vi "H5Lget_val (Soft).vi"(6 "lapl_id":T2, 8 "error in (no error)":errorcluster, 10 "Name":string=".", 11 "Location Ref":T2) -> (0 "error out":errorcluster, 1 "Object Path":string, 3 "Location Ref out":T2, 4 "type":T1 items=["H5L_TYPE_ERROR"=-1, "H5L_TYPE_HARD"=0, "H5L_TYPE_SOFT"=1, "H5L_TYPE_EXTERNAL"=64, "H5L_TYPE_MAX"=255])   [LabVIEW 2017]
doc: "Returns the value of a symbolic link."
uses:
  <vilib>/UPVI/lvhdf5/library.llb/HDF5 Ref.ctl
  <vilib>/UPVI/lvhdf5/link.llb/H5L_type_t.ctl
  <vilib>/UPVI/lvhdf5/error.llb/LVH5EMajorID.ctl
  <vilib>/UPVI/lvhdf5/error.llb/LVH5EMinorID.ctl
  <vilib>/UPVI/lvhdf5/error.llb/H5Epush_enum_enum.vi
panel:
  # "LVHDF5 Toolkit\nCopyright (c) 2005-2013 by Jason D. Sommerville\nCopyright (c) 2014-2015 by UPVI, LLC.\n\nThis use and distribution of this file is governed by the terms found in \nLICENSE.txt distributed with this toolkit and installed at\n <user.lib>\\_lvhdf5\\LICENSE.txt"
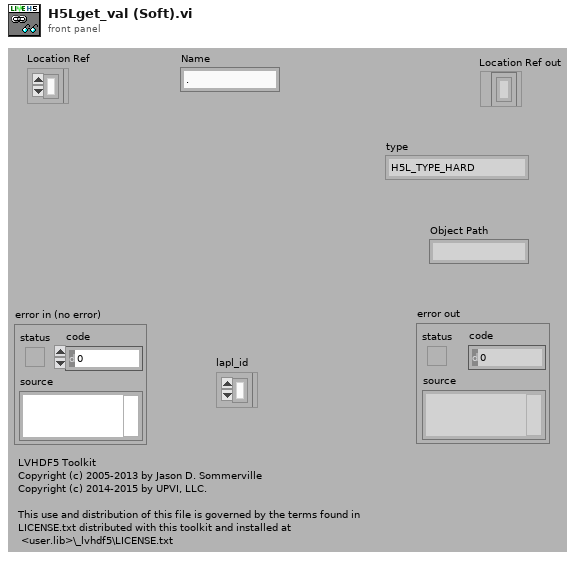
[diagram p1: front panel]
types:
  T1 = typedef "H5L_type_t.ctl" = i32
  T2 = typedef "HDF5 Ref.ctl" = refnum<k1>
  T3 = typedef "LVH5EMinorID.ctl" = string
  T4 = typedef "LVH5EMajorID.ctl" = string
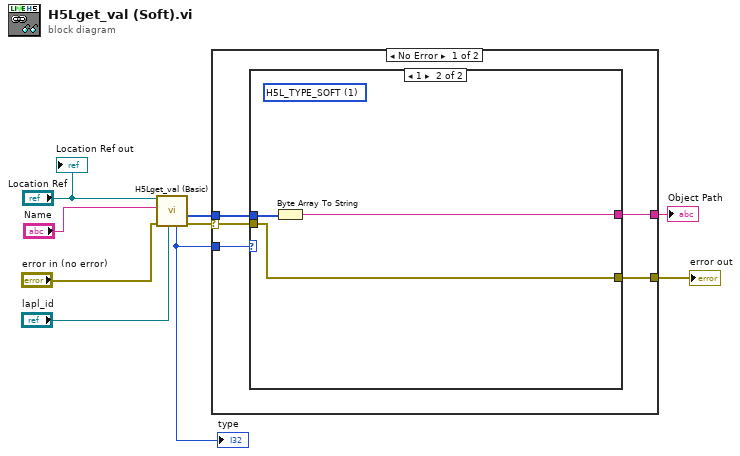
[diagram p0: block diagram]
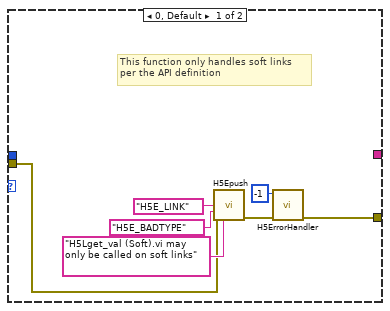
[diagram p2: hidden frame]
diagram:
  n1 = call <vilib>:"H5Lget_val (Basic).vi"("lapl_id"="lapl_id", "error in (no error)"="error in (no error)", "Name"="Name", "Location Ref"="Location Ref") -> ("error out"=w6:errorcluster, "buffer"=w5:u8[], "type"=w1:T1)  [unwired: 4 in, 1 out]
  "type" <- w1
  n2 = case shown="No Error" w6 {
    selector: w6 -> [w12 w25]
    tunnel: w5 -> [w14 _]
    tunnel: [w13 _] -> w3
    tunnel: [w11 w25] -> w4
    tunnel: w1 -> [w10 _]
    frame No Error {
      n3 = case shown="1" w10 {
        tunnel: w14 -> [_ w24]
        tunnel: [_ w23] -> w13
        tunnel: w12 -> [w16 w22]
        tunnel: [w15 w22] -> w11
        frame 0, Default {
          # "This function only handles soft links\nper the API definition"
          n4 = call-poly <vilib>:"H5Epush.vi"("major_id"=T4 "H5E_LINK", "minor_id"=T3 "H5E_BADTYPE", "error in (no error)"=w16, "msg"="H5Lget_val (Soft).vi may only be called on soft links") -> ("error out"=w18:errorcluster)  [unwired: 10 in, 1 out]
          n5 = call <vilib>:"H5ErrorHandler.vi"("error in (no error)"=w18, "herr_t"=-1) -> ("error out"=w15:errorcluster)  [unwired: 3 in, 4 out]
        }
        frame 1 {
          (unwired) T1 1 items=["H5L_TYPE_ERROR"=-1, "H5L_TYPE_HARD"=0, "H5L_TYPE_SOFT"=1, "H5L_TYPE_EXTERNAL"=64, "H5L_TYPE_MAX"=255] ("type")
          n6 = Byte Array To String(unsigned byte array=w24) -> (string=w23:string)
        }
      }
    }
    frame Error {
    }
  }
  "error out" <- w4
  "Object Path" <- w3
  "Location Ref out" <- "Location Ref"
